vi "Close Log File.vi"(8 "error in (no error)":errorcluster, 11 "Logger Interface in":refnum<class "Logger Interface.lvclass">) -> (0 "error out":errorcluster, 3 "Logger Interface out":refnum<class "Logger Interface.lvclass">)   [LabVIEW 2020, in "AIM MIL-STD-1553 Engine.lvlib" / "Implementation.lvlib" / "Word Logging.lvlib" / "Logger Interface.lvclass"]
uses:
  Logger Interface.lvclass
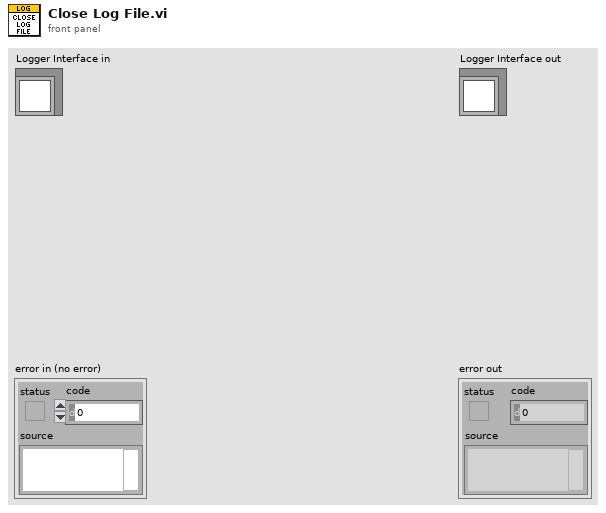
[diagram p1: front panel]
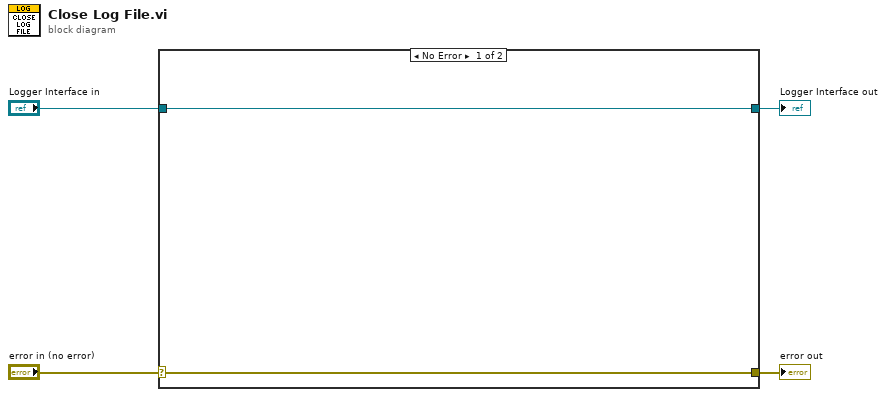
[diagram p0: block diagram]
diagram:
  n1 = case shown="No Error" "error in (no error)" {
    selector: "error in (no error)" -> [w5 w8]
    tunnel: [w5 w8] -> w3
    tunnel: [w6 w7] -> w1
    tunnel: "Logger Interface in" -> [w6 w7]
    frame No Error {
    }
    frame Error {
    }
  }
  "error out" <- w3
  "Logger Interface out" <- w1
